vi "DAQmx.Simulate AI.vi"(8 "error in (no error)":errorcluster, 11 "DAQmx in":refnum<class "DAQmx.lvclass">) -> (0 "error out":errorcluster, 2 "Noisy Signal Graph":waveform(dbl)[](graph), 3 "DAQmx out":refnum<class "DAQmx.lvclass">, 4 "AI time (s)":dbl format="%#_6p")   [LabVIEW 2019, in "DAQmx.lvclass"]
uses:
  Instrument.DAQ/Instrument.DAQ.lvclass/Instrument.DAQ.ctl
  DAQmx.lvclass
panel:
  out "Signal Graph":waveform(dbl)[](graph)
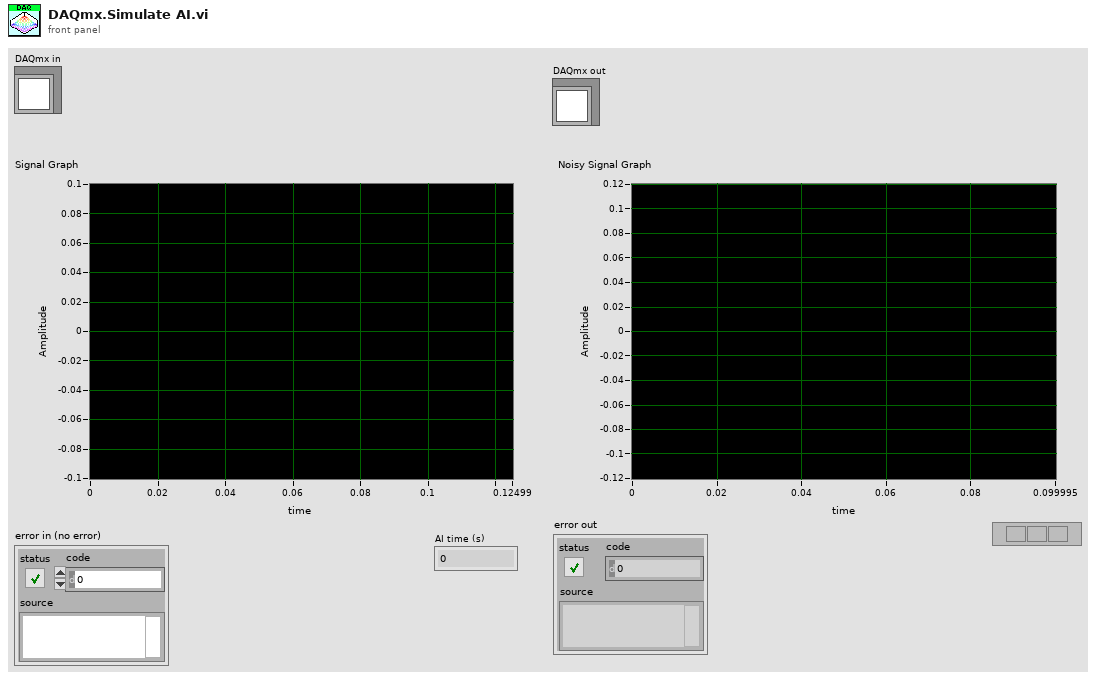
[diagram p1: front panel]
types:
  T1 = typedef "DAQmx.lvclass/DeviceInfo--Cluster.ctl" = cluster{"DeviceName":string, "DevIsSimulated":bool, "DeviceSerialNumber":string, "ProductType":string, "ProductCategory":i32, "ProductNumber":u32, "ChassisNumber":u32, "SlotNumber":u32, "ChassisName":string, "ChassisSerialNumber":string, "DevTemp":dbl, "SelfCal.LastDate/Time":string, "SelfCal.LastTemp":dbl, "calibration due?":bool}
  T2 = typedef "DAQmx.lvclass/DAQ.Config.Timing.Sampling--Cluster.ctl" = cluster{"Fs":dbl, "#s":i32}
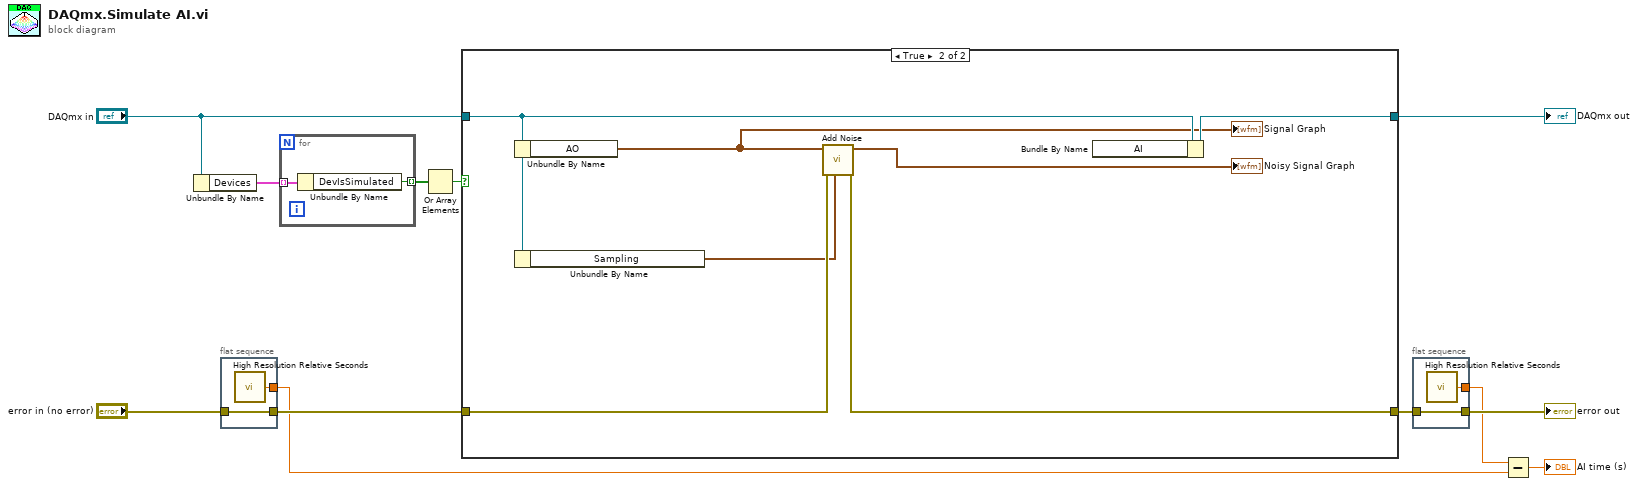
[diagram p0: block diagram]
diagram:
  n1 = Unbundle By Name("DAQmx in") -> ("Devices"=w1:T1[])
  n2 = flat-sequence {
    tunnel: [w14] -> w9
    tunnel: "error in (no error)" -> [w14]
    tunnel: [w13] -> w5
    frame #0 {
      n3 = call <vilib>:"High Resolution Relative Seconds.vi"() -> ("relative seconds"=w13:dbl)
    }
  }
  n4 = for {
    tunnel: w1 -> [w16] mode=indexing
    tunnel: [w15] -> w3 mode=indexing
    n5 = Unbundle By Name(w16) -> ("DevIsSimulated"=w15:bool)
  }
  n6 = Or Array Elements(Boolean array=w3) -> (logical OR=w2:bool)
  n7 = case shown="True" w2 {
    tunnel: "DAQmx in" -> [w18 w23]
    tunnel: [w18 w24] -> w11
    tunnel: w9 -> [w17 w22]
    tunnel: [w17 w25] -> w8
    frame False {
    }
    frame True {
      n8 = Unbundle By Name(w23) -> ("AO"=w20:waveform(dbl)[])
      "Signal Graph" <- w20
      n9 = Unbundle By Name(w23) -> ("Sampling"=w21:T2)
      n10 = call "Add Noise.vi"("Sampling"=w21, "error in (no error)"=w22, "AI []"=w20) -> ("error out"=w25:errorcluster, "AI + Noise"=→"Noisy Signal Graph":waveform(dbl)[])  [unwired: 7 in]
      n11 = Bundle By Name(cluster=w23) -> (w24:refnum<class "DAQmx.lvclass">)  [unwired: 1 in]
    }
  }
  "DAQmx out" <- w11
  n12 = flat-sequence {
    tunnel: [w27] -> w7
    tunnel: w8 -> [w27]
    tunnel: [w26] -> w6
    frame #0 {
      n13 = call <vilib>:"High Resolution Relative Seconds.vi"() -> ("relative seconds"=w26:dbl)
    }
  }
  n14 = Subtract(x=w6, y=w5) -> (x-y=→"AI time (s)":dbl)
  "error out" <- w7
